vi "PrefDialog.vi"(8 "error in (no error)":errorcluster, 11 "SpecAnPlugins.lvlib":refnum<class "Keysight44xx.lvclass">) -> (0 "error out":errorcluster, 1 "Save As?":bool, 2 "Change Occured?":bool=TRUE, 3 "SpecAnPlugins.lvlib":refnum<class "Keysight44xx.lvclass">)   [LabVIEW 2018, in "SpecAnPlugins.lvlib" / "Keysight44xx.lvclass"]
doc: "This VI opens up the modal preference dialog window and allows a user to configure the properties with new values, or keep the existing values from the last time the function was called. The user can also save the new values to a new file name and new type name using the save as button."
uses:
  Keysight44xx.lvclass
  SpecAnBaseClass/Typedefs/Trigger.ctl
  SpecAnBaseClass/Typedefs/Trace.ctl
  SpecAnBaseClass/Typedefs/SweepCoupling.ctl
  SpecAnBaseClass/Typedefs/Level.ctl
  SpecAnBaseClass/Typedefs/Frequency.ctl
  SpecAnBaseClass/Typedefs/Acquisition.ctl
  C:/Program Files (x86)/National Instruments/LabVIEW 2018/user.lib/NIST/BaseClasses/BasePlugin_class/BasePlugin.lvclass
  C:/Users/ico/Documents/Projects/NistPluggableModules/SpecAn/SpecAnPlugins/SpecAnBaseClass/SpecAnBase.lvclass
  TypeDefs/RFBurst.ctl
  TypeDefs/TV.ctl
  SpecAnBaseClass/Typedefs/Markers.ctl
  <userlib>/NIST/BaseClasses/BasePlugin_class/BasePlugin.lvclass/BasePlugin.ctl
  <userlib>/NIST/BaseClasses/BasePlugin_class/Accessors/Read PluginIniFilePath.vi
  <userlib>/NIST/BaseClasses/BasePlugin_class/Accessors/Write PluginIniFilePath.vi
  <vilib>/Utility/config.llb/NI_LVConfig.lvlib
  SpecAnBaseClass/SpecAnBase.lvclass
panel:
  in  "Tab Control":T1(tab)
  in  "Acquisition":T2={"Handle"="who", "Connected"=FALSE, "Enabled"=TRUE, "SweepModeContinuous"=TRUE, "NumberOfSweeps"=1, "DetectorTypeAuto"=TRUE, "DetectorType"=2, "VerticalScale"=1, "MaximumTime(seconds)"=1.0} {"VerticalScale" items=["Linear", "Logarithmic"]; "DetectorType" items=["AutoPeak", "Average", "MaximumPeak", "MinimumPeak", "Sample", "RMS"]}
  in  "Frequency":T3={"FrequencyStart"=5000.0, "FrequencyStop"=10000.0, "FrequencyOffset"=0.0}
  in  "Level":T4={"InputImpedance"=50.0, "AttenuationAuto"=FALSE, "ReferenceLevel"=0.0, "Attenuation"=0.0, "ReferenceLevelOffset"=0.0, "amplitude units (dBm)"=1} {"amplitude units (dBm)" items=["dBm"=1, "dBmV"=2, "dBuV"=3, "dBuA"=1001, "Volt"=4, "Watt"=5, "Amper"=1002]}
  in  "SweepCoupling":T5={"ResolutionBandwidth"=3000000.0, "ResolutionBandwidthAuto"=TRUE, "SweepTime"=0.004, "VideoBandwidth"=300000.0, "VideoBandwidthAuto"=TRUE, "SweepTimeAuto"=TRUE}
  in  "Trace":T6=[{"TraceName"="TRACE1", "TraceSize"=200, "TraceType"=1}] {"TraceType" items=["Clear Write"=1, "Maximum Hold"=2, "Minimum Hold"=3, "View"=4, "Store"=5, "Video Average"=6]}
  in  "RF Burst":T7={"Frequency Selectivity (OFF)"=FALSE, "Trigger Level Type (Absolute)"=1, "Narrow Pulse Discriminator (OFF)"=FALSE} {"Trigger Level Type (Absolute)" items=["Absolute"=1, "Relative"=2]}
  in  "Trigger":T8={"TriggerLevel"=0.0, "TriggerSlope"=1, "Trigger Source"=2} {"Trigger Source" items=["External"=1, "Immediate"=2, "AC Line"=4, "Video"=5, "TV"=1001, "RF Burst"=1002]; "TriggerSlope" items=["Positive"=1, "Negative"=2]}
  in  "TV":T9={"Monitor Enabled (OFF)"=FALSE, "SynchronizeSweep"=FALSE, "SynchronizationLineNumber"=0, "TV Field (Any Field)"=3, "TV Signal Format (NTSC-M)"=1, "Trigger Source (Spectrum Analyzer)"=2} {"Trigger Source (Spectrum Analyzer)" items=["External"=1, "Spectrum Analyzer"=2]; "TV Signal Format (NTSC-M)" items=["NTSC-M"=1, "NTSC-Japan"=2, "PAL-M"=3, "PAL-B,D,G,H,I"=4, "PAL-N"=5, "PAL-N Combin"=6, "SECAM-L"=7]; "TV Field (Any Field)" items=["Field 1"=1, "Field 2"=2, "Any Field"=3]}
  in  "Marker":T10={"MarkerEnabled"=TRUE, "MarkerThreshold"=0.0, "PeakExcursion"=0.0, "SignalTrackEnabled"=FALSE, "MarkerPosition"=7500.0, "Instrument Setting (Frequency Center)"=3, "Marker search (Minimum)"=2, "ActiveMarker"="MARKER1", "MarkerFrequencyCounter"=FALSE, "FrequencyCounterResolution"=0.0} {"Marker search (Minimum)" items=["Highest"=1, "Next Peak"=3, "Next Peak Left"=4, "Next Peak Right"=5, "Minimum"=2]; "Instrument Setting (Frequency Center)" items=["Frequency Start"=3, "Frequency Stop"=4, "Frequency Center"=1, "Frequency Span"=2, "Reference Level"=5]}
  in  "btnSave":bool
  in  "btnSaveAs":bool
  in  "btnCancel":bool
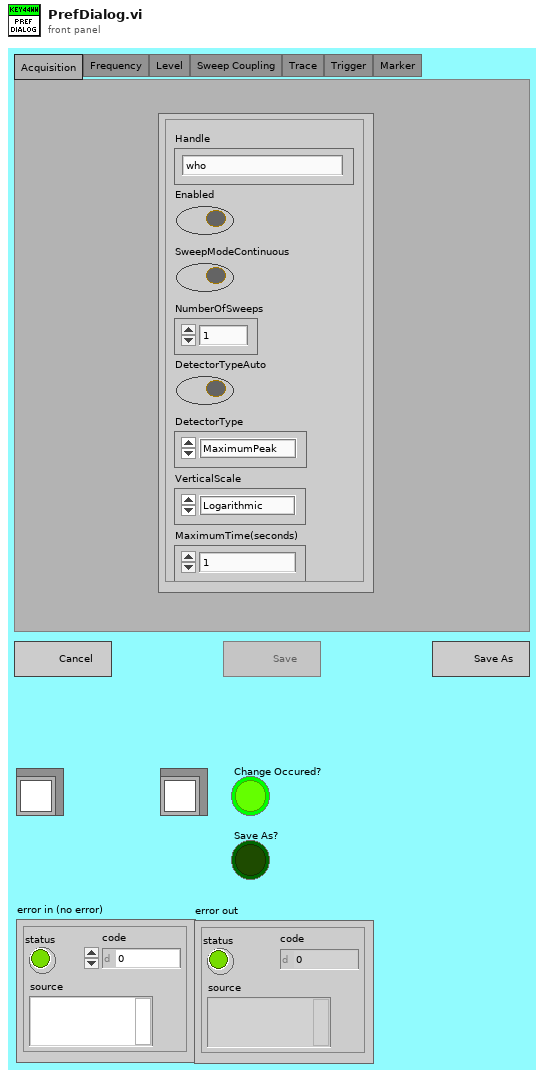
[diagram p1: front panel]
types:
  T1 = enum32{"Acquisition", "Frequency", "Level", "Sweep Coupling", "Trace", "Trigger", "Marker"}
  T2 = typedef "SpecAnPlugins.lvlib/SpecAnBase.lvclass/Acquisition.ctl" = cluster{"Handle":string, "Connected":bool, "Enabled":bool, "SweepModeContinuous":bool, "NumberOfSweeps":i32, "DetectorTypeAuto":bool, "DetectorType":i32, "VerticalScale":i32, "MaximumTime(seconds)":dbl}
  T3 = typedef "SpecAnPlugins.lvlib/SpecAnBase.lvclass/Frequency.ctl" = cluster{"FrequencyStart":dbl, "FrequencyStop":dbl, "FrequencyOffset":dbl}
  T4 = typedef "SpecAnPlugins.lvlib/SpecAnBase.lvclass/Level.ctl" = cluster{"InputImpedance":dbl, "AttenuationAuto":bool, "ReferenceLevel":dbl, "Attenuation":dbl, "ReferenceLevelOffset":dbl, "amplitude units (dBm)":i32}
  T5 = typedef "SpecAnPlugins.lvlib/SpecAnBase.lvclass/SweepCoupling.ctl" = cluster{"ResolutionBandwidth":dbl, "ResolutionBandwidthAuto":bool, "SweepTime":dbl, "VideoBandwidth":dbl, "VideoBandwidthAuto":bool, "SweepTimeAuto":bool}
  T6 = typedef "SpecAnPlugins.lvlib/SpecAnBase.lvclass/Trace.ctl" = cluster{"TraceName":string, "TraceSize":i32, "TraceType":i32}[]
  T7 = typedef "SpecAnPlugins.lvlib/Keysight44xx.lvclass/RFBurst.ctl" = cluster{"Frequency Selectivity (OFF)":bool, "Trigger Level Type (Absolute)":i32, "Narrow Pulse Discriminator (OFF)":bool}
  T8 = typedef "SpecAnPlugins.lvlib/SpecAnBase.lvclass/Trigger.ctl" = cluster{"TriggerLevel":dbl, "TriggerSlope":i32, "Trigger Source":i32}
  T9 = typedef "SpecAnPlugins.lvlib/Keysight44xx.lvclass/TV.ctl" = cluster{"Monitor Enabled (OFF)":bool, "SynchronizeSweep":bool, "SynchronizationLineNumber":i32, "TV Field (Any Field)":i32, "TV Signal Format (NTSC-M)":i32, "Trigger Source (Spectrum Analyzer)":i32}
  T10 = typedef "SpecAnPlugins.lvlib/SpecAnBase.lvclass/Markers.ctl" = cluster{"MarkerEnabled":bool, "MarkerThreshold":dbl, "PeakExcursion":dbl, "SignalTrackEnabled":bool, "MarkerPosition":dbl, "Instrument Setting (Frequency Center)":i32, "Marker search (Minimum)":i32, "ActiveMarker":string, "MarkerFrequencyCounter":bool, "FrequencyCounterResolution":dbl}
  T11 = enum32{"Invalid", "Default", "Floating", "Floating/Auto-Hide", "Modal"}
  T12 = enum8{"Enabled", "Disabled", "Disabled and Grayed Out"}
  T13 = typedef "NI_LVConfig.lvlib/Config Data RefNum.ctl" = refnum<k1>
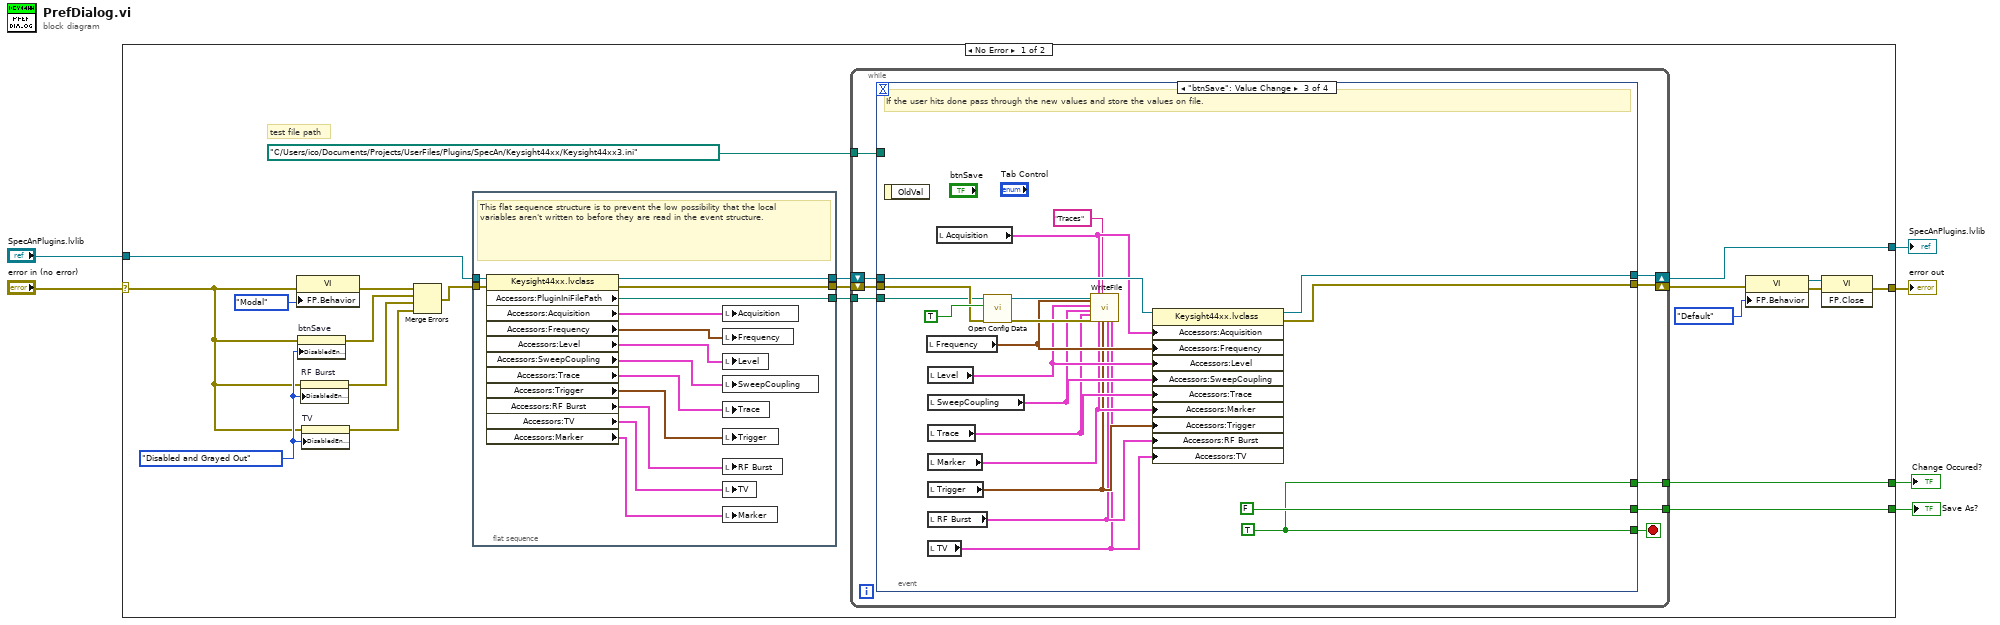
[diagram p0: block diagram]
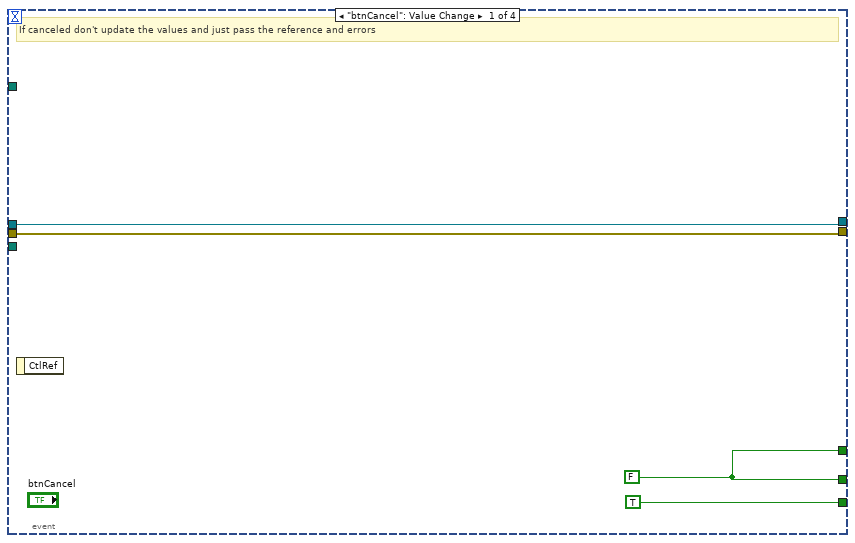
[diagram p2: hidden frame]
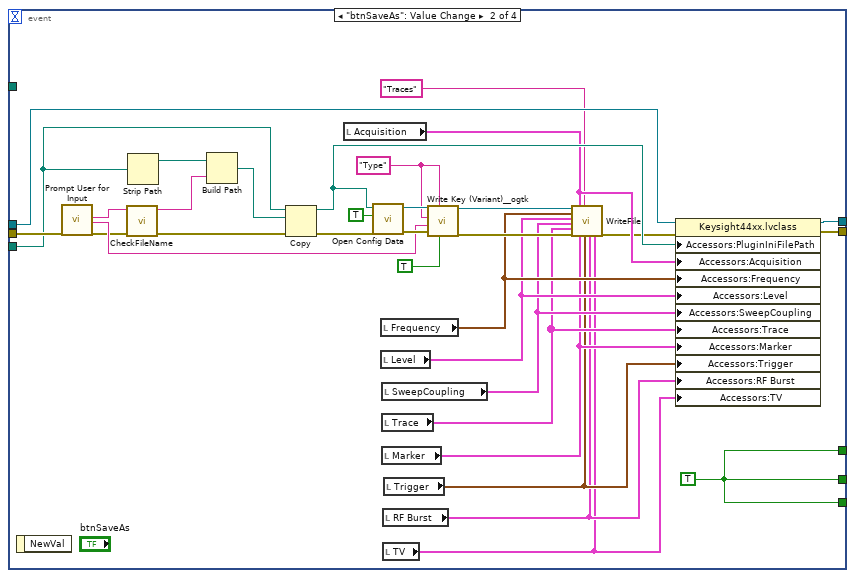
[diagram p3: hidden frame]
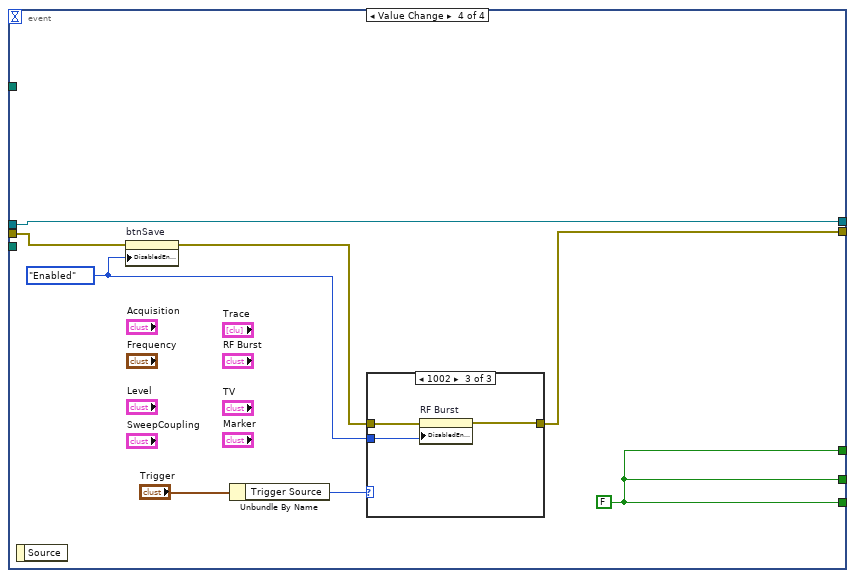
[diagram p4: hidden frame]
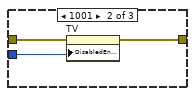
[diagram p6: hidden frame]
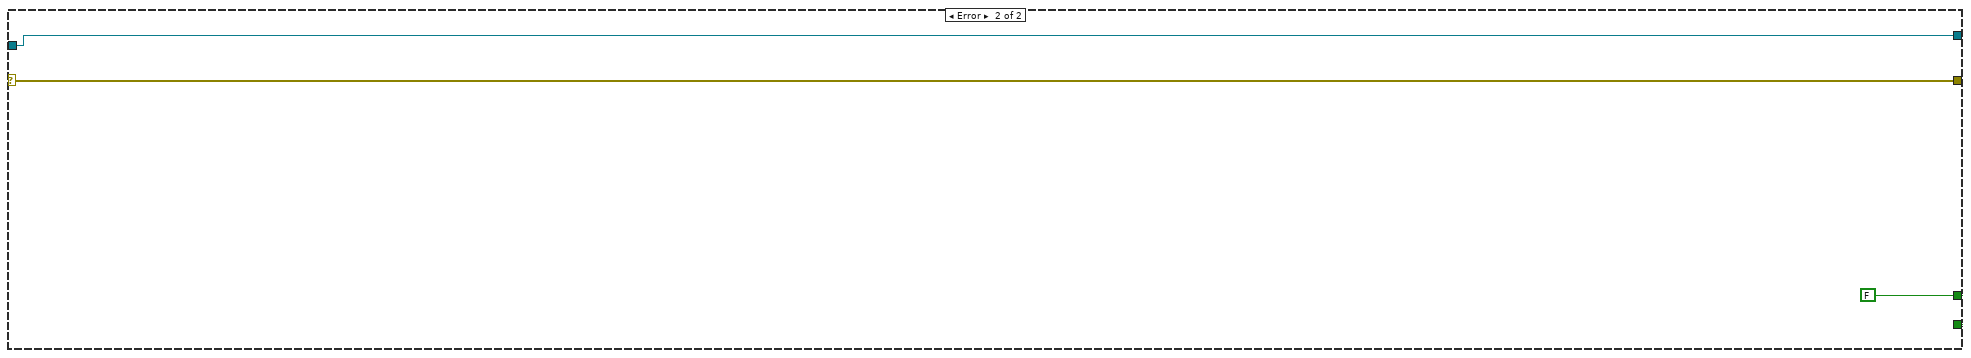
[diagram p7: hidden frame]
diagram:
  n1 = case shown="No Error" "error in (no error)" {
    selector: "error in (no error)" -> [w13 w124]
    tunnel: [w24 w124] -> w1
    tunnel: "SpecAnPlugins.lvlib" -> [w22 w123]
    tunnel: [w18 w123] -> w4
    tunnel: [w16 w125] -> w3
    tunnel: [w15 w125] -> w2
    frame No Error {
      w14 = T12."Disabled and Grayed Out" ("Disabled")
      # "test file path"
      n2 = property class="VI"(error in=w13, "FP.Behavior"=T11."Modal" ("Front Panel Window:Behavior")) -> (error out=w12:errorcluster)  [unwired: 1 in, 1 out]
      n3 = property on="btnSave" class="Bool"(error in=w13, "DisabledEnum"=w14) -> (error out=w10:errorcluster)  [unwired: 1 in, 1 out]
      n4 = property on="RF Burst" class="Clust (strict)"(error in=w13, "DisabledEnum"=w14) -> (error out=w9:errorcluster)  [unwired: 1 in, 1 out]
      n5 = property on="TV" class="Clust (strict)"(error in=w13, "DisabledEnum"=w14) -> (error out=w8:errorcluster)  [unwired: 1 in, 1 out]
      n6 = Merge Errors(w12, w10, w9, w8) -> (w11:errorcluster)
      n7 = flat-sequence {
        tunnel: w22 -> [w41]
        tunnel: w11 -> [w40]
        tunnel: [w39] -> w21
        tunnel: [w38] -> w20
        tunnel: [w37] -> w19
        frame #0 {
          # "This flat sequence structure is to prevent the low possibility that the local variables aren't written to before they are read in the event structure."
          n8 = property class="Keysight44xx.lvclass"(reference=w41, error in=w40) -> (reference out=w38:refnum<class "Keysight44xx.lvclass">, error out=w39:errorcluster, "Accessors:PluginIniFilePath"=w37:path, "Accessors:Acquisition"=w36:T2, "Accessors:Frequency"=w35:T3, "Accessors:Level"=w34:T4, "Accessors:SweepCoupling"=w33:T5, "Accessors:Trace"=w32:T6, "Accessors:Trigger"=w31:T8, "Accessors:RF Burst"=w30:T7, "Accessors:TV"=w29:T9, "Accessors:Marker"=w28:T10)
          n9 = local write "Acquisition"(w36) -> ()
          n10 = local write "Frequency"(w35) -> ()
          n11 = local write "Level"(w34) -> ()
          n12 = local write "SweepCoupling"(w33) -> ()
          n13 = local write "Trace"(w32) -> ()
          n14 = local write "Trigger"(w31) -> ()
          n15 = local write "RF Burst"(w30) -> ()
          n16 = local write "TV"(w29) -> ()
          n17 = local write "Marker"(w28) -> ()
        }
      }
      n18 = while {
        tunnel: w19 -> [w48]
        shift-right: [w46] -> w17
        shift-left: w21 -> [w50]
        shift-right: [w47] -> w18
        shift-left: w20 -> [w49]
        tunnel: [w44] -> w15
        tunnel: [w43] -> w16
        tunnel: path "C:/Users/ico/Documents/Projects/UserFiles/Plugins/SpecAn/Keysight44xx/Keysight44xx3.ini" ("Accessors:PluginIniFilePath") -> [w42]
        stop <- w45 stop-if-true
        n19 = event shown="[2] \"btnSave\": Value Change" {
          selector: _ -> [_ _ _ _]
          dyn-events: _ -> [_ _ _ _]
          timeout: _ -> [_ _ _ _]
          tunnel: w50 -> [w53 w85 w103 w114]
          tunnel: w49 -> [w54 w77 w107 w115]
          tunnel: w48 -> [_ w68 w100 _]
          tunnel: [w54 w87 w106 w115] -> w47
          tunnel: [w53 w86 w105 w108] -> w46
          tunnel: [TRUE w71 w101 w113] -> w45
          tunnel: [w51 w71 FALSE w113] -> w44
          tunnel: [w51 w71 w101 w113] -> w43
          tunnel: w42 -> [_ _ _ _]
          event "btnCancel": Value Change {
            w51 = FALSE
            # "If canceled don't update the values and just pass the reference and errors"
            n20 = event-data() -> ()  [unwired: 1 in, 1 out]
          }
          event "btnSaveAs": Value Change {
            w74 = "Type" ("section")
            w71 = TRUE
            n21 = event-data() -> ()  [unwired: 1 in, 1 out]
            n22 = call "Prompt User for Input"("error in (no error)"=w85) -> ("File Name"=w81:string, "PluginType"=w73:string, "error out"=w70:errorcluster)  [unwired: 15 in, 1 out]
            n23 = call "CheckFileName.vi"("Error In"=w70, "File Name in"=w81) -> ("Error Out"=w69:errorcluster, "File Name out"=w82:string)  [unwired: 8 in]
            n24 = Strip Path(path=w68) -> (stripped path=w84:path)  [unwired: 1 out]
            n25 = Build Path(base path=w84, name or relative path=w82) -> (appended path=w83:path)
            n26 = Copy(8:w69, 10:w83, 11:w68) -> (0:w79:errorcluster, 3:w78:path)  [unwired: 2 in, 1 out]
            n27 = local read "Acquisition"() -> (w67:T2)
            n28 = call <vilib>:"Open Config Data.vi"("error in (no error)"=w79, "create file if necessary (T)"=TRUE, "configuration file path"=w78) -> ("error out"=w76:errorcluster, "refnum"=w75:T13)  [unwired: 6 in, 1 out]
            n29 = local read "Frequency"() -> (w63:T3)
            n30 = local read "Level"() -> (w62:T4)
            n31 = local read "SweepCoupling"() -> (w61:T5)
            n32 = local read "Trace"() -> (w60:T6)
            n33 = local read "Marker"() -> (w59:T10)
            n34 = local read "RF Burst"() -> (w57:T7)
            n35 = local read "TV"() -> (w56:T9)
            n36 = local read "Trigger"() -> (w58:T8)
            n37 = call <userlib>:"Write Key (Variant)__ogtk.vi"("write raw string? (F)"=TRUE, "section"=w74, "error in (no error)"=w76, "key-value"=w73, "key (optional)"=w74, "refnum"=w75) -> ("error out"=w64:errorcluster, "refnum out"=w66:T13)  [unwired: 4 in]
            n38 = call "WriteFile.vi"("refnum"=w66, "Frequency"=w63, "Level"=w62, "SweepCoupling"=w61, "Trace"=w60, "error in (no error)"=w64, "Acquisition"=w67, "Marker"=w59, "section"="Traces", "Trigger"=w58, "RF Burst"=w57, "TV"=w56) -> ("error out"=w55:errorcluster)  [unwired: 7 in]
            n39 = property class="Keysight44xx.lvclass"(reference=w77, error in=w55, "Accessors:PluginIniFilePath"=w78, "Accessors:Acquisition"=w67, "Accessors:Frequency"=w63, "Accessors:Level"=w62, "Accessors:SweepCoupling"=w61, "Accessors:Trace"=w60, "Accessors:Marker"=w59, "Accessors:Trigger"=w58, "Accessors:RF Burst"=w57, "Accessors:TV"=w56) -> (reference out=w87:refnum<class "Keysight44xx.lvclass">, error out=w86:errorcluster)
          }
          event "btnSave": Value Change {
            w101 = TRUE
            # "If the user hits done pass through the new values and store the values on file."
            n40 = event-data() -> ()  [unwired: 1 in, 1 out]
            n41 = local read "Frequency"() -> (w95:T3)
            n42 = local read "Level"() -> (w94:T4)
            n43 = local read "SweepCoupling"() -> (w93:T5)
            n44 = local read "Trace"() -> (w92:T6)
            n45 = local read "Marker"() -> (w91:T10)
            n46 = local read "Trigger"() -> (w90:T8)
            n47 = local read "RF Burst"() -> (w89:T7)
            n48 = local read "TV"() -> (w88:T9)
            n49 = local read "Acquisition"() -> (w97:T2)
            n50 = call <vilib>:"Open Config Data.vi"("error in (no error)"=w103, "create file if necessary (T)"=TRUE, "configuration file path"=w100) -> ("error out"=w98:errorcluster, "refnum"=w99:T13)  [unwired: 6 in, 1 out]
            n51 = call "WriteFile.vi"("refnum"=w99, "Frequency"=w95, "Level"=w94, "SweepCoupling"=w93, "Trace"=w92, "error in (no error)"=w98, "Acquisition"=w97, "Marker"=w91, "section"="Traces", "Trigger"=w90, "RF Burst"=w89, "TV"=w88) -> ()  [unwired: 7 in, 1 out]
            n52 = property class="Keysight44xx.lvclass"(reference=w107, "Accessors:Acquisition"=w97, "Accessors:Frequency"=w95, "Accessors:Level"=w94, "Accessors:SweepCoupling"=w93, "Accessors:Trace"=w92, "Accessors:Marker"=w91, "Accessors:Trigger"=w90, "Accessors:RF Burst"=w89, "Accessors:TV"=w88) -> (reference out=w106:refnum<class "Keysight44xx.lvclass">, error out=w105:errorcluster)  [unwired: 1 in]
          }
          event Value Change {
            w113 = FALSE
            w109 = T12."Enabled" ("Disabled")
            n53 = event-data() -> ()  [unwired: 1 in, 1 out]
            n54 = property on="btnSave" class="Bool"(error in=w114, "DisabledEnum"=w109) -> (error out=w110:errorcluster)  [unwired: 1 in, 1 out]
            n55 = Unbundle By Name("Trigger") -> ("Trigger Source"=w111:i32)
            n56 = case shown="1002" w111 {
              tunnel: w110 -> [w116 w119 w122]
              tunnel: w109 -> [_ w117 w121]
              tunnel: [w116 w118 w120] -> w108
              frame 1, Default {
              }
              frame 1001 {
                n57 = property on="TV" class="Clust (strict)"(error in=w119, "DisabledEnum"=w117) -> (error out=w118:errorcluster)  [unwired: 1 in, 1 out]
              }
              frame 1002 {
                n58 = property on="RF Burst" class="Clust (strict)"(error in=w122, "DisabledEnum"=w121) -> (error out=w120:errorcluster)  [unwired: 1 in, 1 out]
              }
            }
          }
        }
      }
      n59 = property class="VI"(error in=w17, "FP.Behavior"=T11."Default" ("Front Panel Window:Behavior")) -> (reference out=w23:refnum<vi>, error out=w26:errorcluster)  [unwired: 1 in]
      n60 = invoke class="VI" method="FP.Close"(reference=w23, error in=w26) -> (error out=w24:errorcluster)  [unwired: 1 in, 2 out]
    }
    frame Error {
      w125 = FALSE
    }
  }
  "error out" <- w1
  "SpecAnPlugins.lvlib" <- w4
  "Change Occured?" <- w3
  "Save As?" <- w2
